vi "Retrieve Process from App.vi"(8 "error in (no error)":errorcluster, 10 "String":string, 11 "Application In":refnum<class "Application.lvclass">) -> (0 "error out":errorcluster, 2 "Process":refnum<class "Process.lvclass">, 3 "Application Out":refnum<class "Application.lvclass">)   [LabVIEW 2020, in "Application.lvclass"]
uses:
  Application.lvclass
  C:/Users/anton/Documents/GitHub/Triarc-Framework/source/Framework/Process/Process.lvclass
  Process/Process.lvclass
  Process/Process.lvclass/Process.ctl
  Application.lvclass/Application.ctl
  Process/Public/Lifecycle/Get Lifecycle State.vi
  Process/Private/SubVIs/Enqueue Request Message.vi
  <vilib>/Utility/error.llb/Clear Errors.vi
  <vilib>/Utility/error.llb/Error Cluster From Error Code.vi
  Process/Private/SubVIs/Wait for Response Message.vi
  Process/Public/Read Name.vi
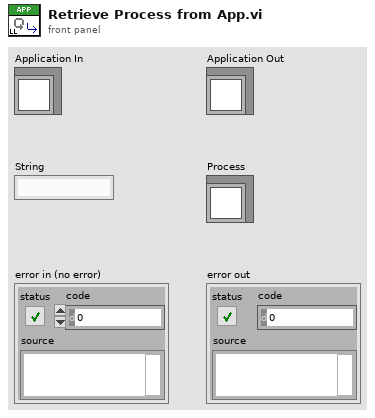
[diagram p1: front panel]
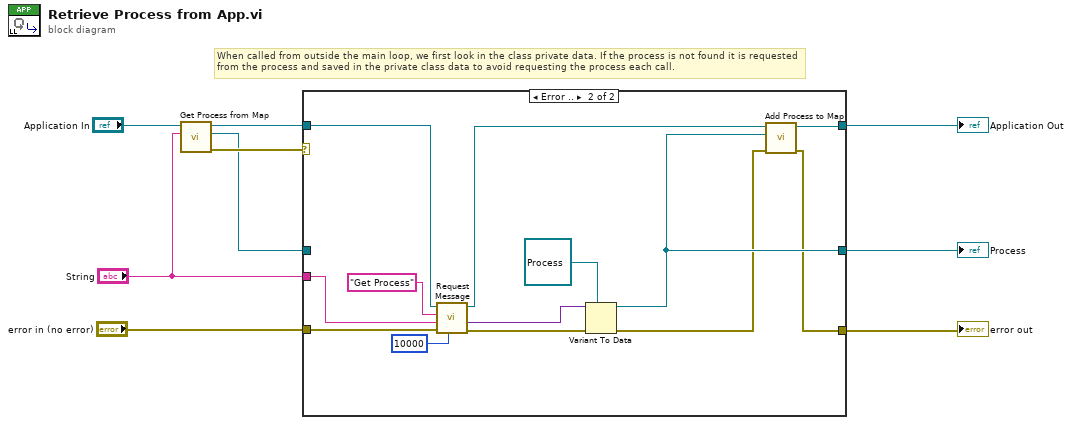
[diagram p0: block diagram]
diagram:
  # "When called from outside the main loop, we first look in the class private data. If the process is not found it is requested from the process and saved in the private class data to avoid requesting the process each call."
  n1 = call "Get Process from Map.vi"("Process Name"="String", "Application In"="Application In") -> ("error out"=w3:errorcluster, "Process"=w2:refnum<class "Process.lvclass">, "Application Out"=w4:refnum<class "Application.lvclass">)  [unwired: 7 in]
  n2 = case shown="Error .." w3 {
    tunnel: [w12 w13] -> w8
    tunnel: [w10 w15] -> w6
    tunnel: "error in (no error)" -> [w12 w21]
    tunnel: w4 -> [w11 w20]
    tunnel: "String" -> [_ w19]
    tunnel: w2 -> [w10 _]
    tunnel: [w11 w16] -> w7
    frame No Error {
      # "Or we have not started process"
      # "Or we are in process loop"
      # "Process has been requested before and is found in current object"
    }
    frame Error {
      n3 = call "Request Message.vi"("timeout in ms (-1)"=10000, "error in (no error)"=w21, "Request Message Data"=w19, "Request Message"="Get Process", "Process In"=w20) -> ("error out"=w25:errorcluster, "Response Message Data"=w23:variant, "Process Out"=w17:refnum<class "Application.lvclass">)  [unwired: 2 in, 2 out]
      n4 = Variant To Data(error in=w25, type=refnum<class "Process.lvclass"> refnum ("Rig Process"), Variant=w23) -> (data=w15:refnum<class "Process.lvclass">, error out=w14:errorcluster)
      n5 = call "Add Process to Map.vi"("error in (no error)"=w14, "Process Out"=w15, "Application In"=w17) -> ("error out"=w13:errorcluster, "Application Out"=w16:refnum<class "Application.lvclass">)  [unwired: 7 in]
    }
  }
  "error out" <- w8
  "Application Out" <- w7
  "Process" <- w6
